vi "%Acquired.vi"(8 "error in (no error)":errorcluster, 11 "CCD in":refnum<class "CCD.lvclass">) -> (0 "error out":errorcluster, 3 "CCD out":refnum<class "CCD.lvclass">)   [LabVIEW 2018, in "CCD.lvclass"]
uses:
  CCD.lvclass
  CCD.lvclass/CCD.ctl
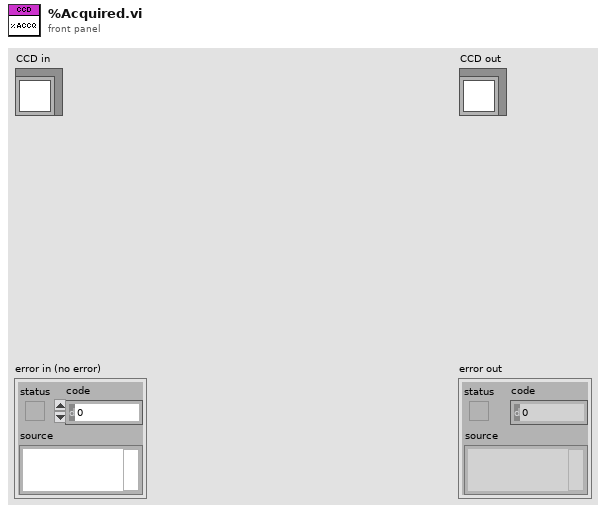
[diagram p1: front panel]
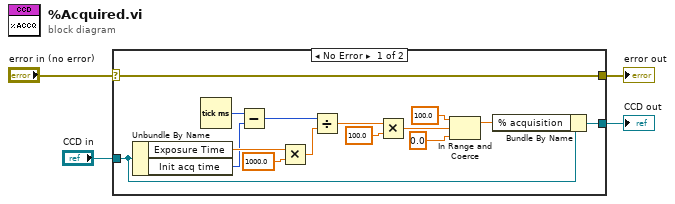
[diagram p0: block diagram]
diagram:
  n1 = case shown="No Error" "error in (no error)" {
    selector: "error in (no error)" -> [w5 w21]
    tunnel: [w5 w21] -> w1
    tunnel: [w7 w20] -> w2
    tunnel: "CCD in" -> [w8 w20]
    frame No Error {
      n2 = Unbundle By Name(w8) -> ("Exposure Time"=w19:dbl, "Init acq time"=w9:u32)
      n3 = Tick Count (ms)() -> (millisecond timer value=w10:u32)
      n4 = Subtract(x=w10, y=w9) -> (x-y=w16:u32)
      n5 = Multiply(x=w19, y=1000.0) -> (x*y=w17:dbl)
      n6 = Divide(x=w16, y=w17) -> (x/y=w15:dbl)
      n7 = Multiply(x=w15, y=100.0) -> (x*y=w11:dbl)
      n8 = In Range and Coerce(upper limit=100.0 ("y"), x=w11, lower limit=0.0) -> (coerced(x)=w6:dbl)  [unwired: 1 out]
      n9 = Bundle By Name(cluster=w8, "% acquisition"=w6) -> (w7:refnum<class "CCD.lvclass">)
    }
    frame Error {
    }
  }
  "error out" <- w1
  "CCD out" <- w2
